vi "Create G-CLI Script lvBuild Installer.vi"(8 "error in (no error)":errorcluster, 11 "PostBuildSupport in":refnum<class "PostBuildSupport.lvclass">) -> (0 "error out":errorcluster, 2 "command":string, 3 "PostBuildSupport out":refnum<class "PostBuildSupport.lvclass">)   [LabVIEW 2019, in "PostBuildSupport.lvclass"]
uses:
  PostBuildSupport.lvclass
  PostBuildSupport.lvclass/PostBuildSupport.ctl
  VIPM/VIPM.lvlib
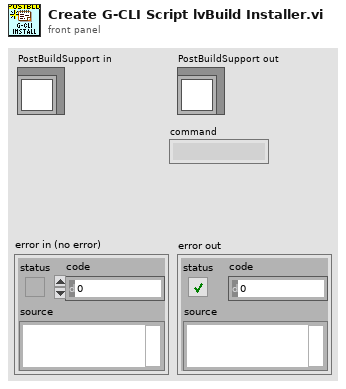
[diagram p1: front panel]
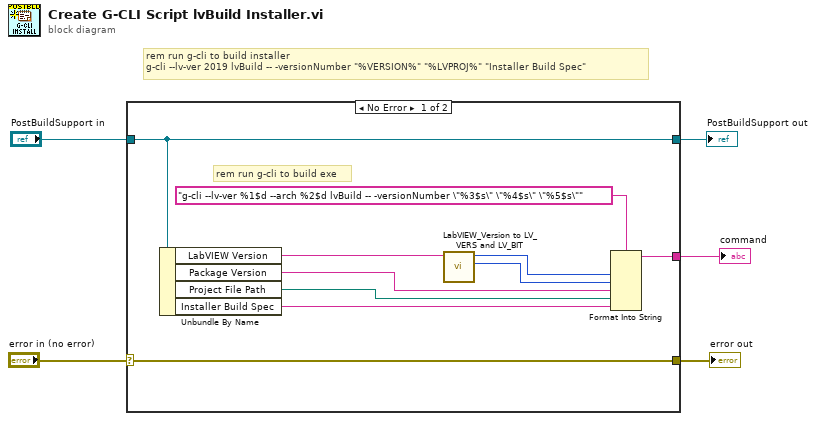
[diagram p0: block diagram]
diagram:
  # "rem run g-cli to build installer\ng-cli --lv-ver 2019 lvBuild -- -versionNumber \"%VERSION%\" \"%LVPROJ%\" \"Installer Build Spec\""
  n1 = case shown="No Error" "error in (no error)" {
    selector: "error in (no error)" -> [w10 w17]
    tunnel: "PostBuildSupport in" -> [w15 w16]
    tunnel: [w10 w17] -> w3
    tunnel: [w15 w16] -> w2
    tunnel: [w11 _] -> w1
    frame No Error {
      # "rem run g-cli to build exe"
      n2 = Unbundle By Name(w15) -> ("LabVIEW Version"=w8:string, "Package Version"=w12:string, "Project File Path"=w6:path, "Installer Build Spec"=w13:string)
      n3 = call "LabVIEW_Version to LV_VERS and LV_BIT.vi"("Package_LabVIEW_Version"=w8) -> ("LV_BIT"=w9:u32, "LV_VER"=w7:u32)  [unwired: 9 in]
      n4 = Format Into String(format string="g-cli --lv-ver %1$d --arch %2$d lvBuild -- -versionNumber \"%3$s\" \"%4$s\" \"%5$s\"", w7, w9, w12, w6, w13) -> (resulting string=w11:string)  [unwired: 2 in, 1 out]
    }
    frame Error {
    }
  }
  "error out" <- w3
  "PostBuildSupport out" <- w2
  "command" <- w1
